vi "Create DGML.vi"(8 "error in (no error)":errorcluster, 10 "Array":T1[](array[typedef]), 11 "Create Unowned Container?":bool) -> (0 "error out":errorcluster, 2 "DGML File":string)   [LabVIEW 2018, in "Shared Dependencies.lvlib"]
uses:
  Name and Dependency processing/Name - Dep Cluster.ctl
  Shared Dependencies.lvlib
  DGML Creation/DGML creation.lvlib
  Name and Dependency processing/Name and Dependency Processing.lvlib
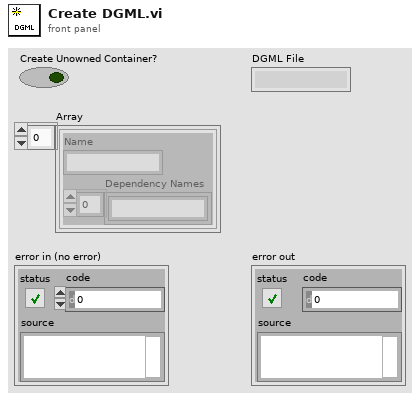
[diagram p1: front panel]
types:
  T1 = typedef "Name and Dependency Processing.lvlib/Name - Dep Cluster.ctl" = cluster{"Name":string, "Dependency Names":string[]}
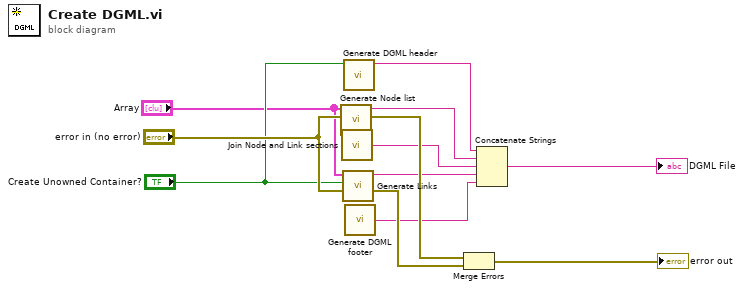
[diagram p0: block diagram]
diagram:
  n1 = call "Generate Node list.vi"("error in"="error in (no error)", "Node-Dep Cluster"="Array") -> ("error out"=w7:errorcluster, "Node List"=w10:string)  [unwired: 8 in]
  n2 = call "Join Node and Link sections.vi"() -> ("string"=w1:string)
  n3 = call "Generate Links.vi"("error in (no error)"="error in (no error)", "Create Unowned Container?"="Create Unowned Container?", "Name-Dep array"="Array") -> ("error out"=w9:errorcluster, "String"=w2:string)  [unwired: 7 in]
  n4 = call "Generate DGML header.vi"("Create Unowned Container?"="Create Unowned Container?") -> ("String"=w11:string)  [unwired: 10 in]
  n5 = call "Generate DGML footer.vi"() -> ("string"=w3:string)
  n6 = Merge Errors(w7, w9) -> (→"error out":errorcluster)
  n7 = Concatenate Strings(w11, w10, w1, w2, w3) -> (→"DGML File":string)
